vi "XW_file_info.vi"(0 "Instrument type":T1=enum."Cross wire angle", 1 "Ch No":i16) -> (2 "Filename":path, 3 "resulting string":string, 4 "File Exists?":bool)   [LabVIEW 2010]
uses:
  Controls/Cal_Inst_type.ctl
  Globals/Constants_global.vi
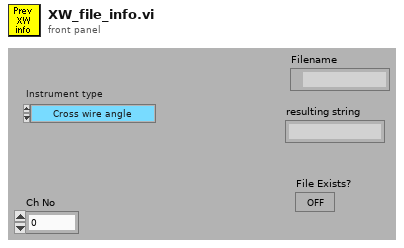
[diagram p1: front panel]
types:
  T1 = typedef "Cal_Inst_type.ctl" = enum16{"Propeller anemometer", "Pressure Transducer", "Hot wire", "Cross wire velocity", "Cross wire angle", "Generic Linear", "Generic Polynomial", "Generic BackPoly", "Fast FID", "Thermocouple", "Cold wire", "Pulsed Wire"}
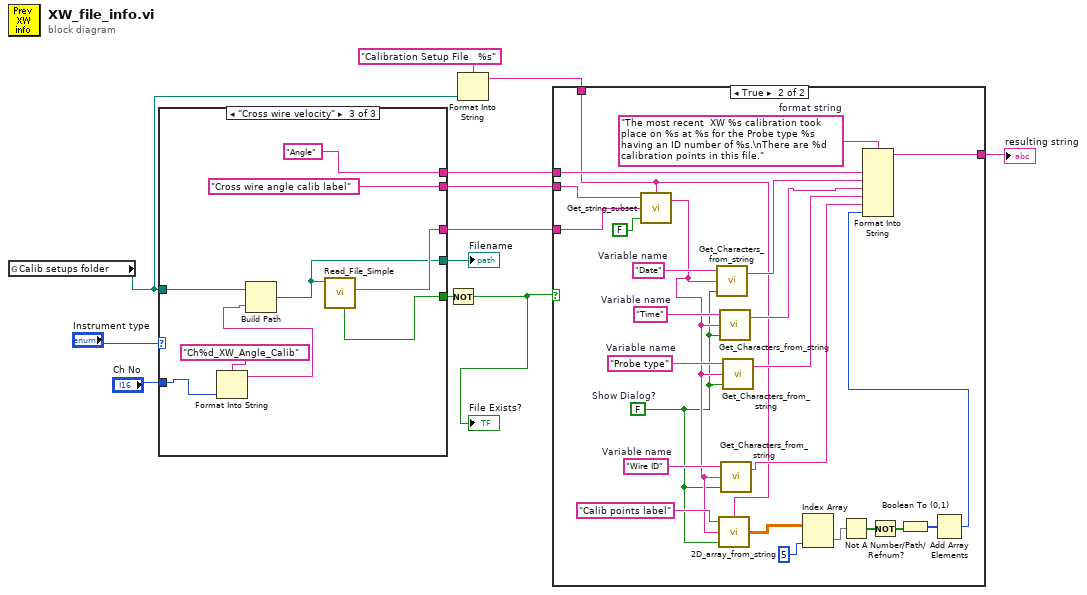
[diagram p0: block diagram]
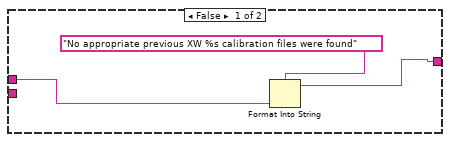
[diagram p2: hidden frame]
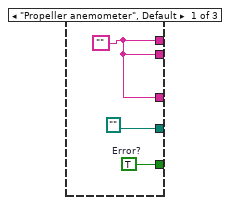
[diagram p3: hidden frame]
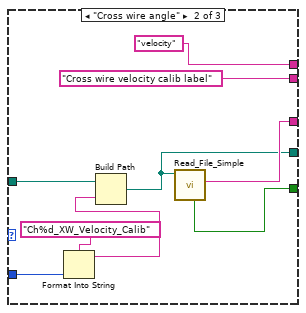
[diagram p4: hidden frame]
diagram:
  n1 = global read "Constants_global.vi" "Calib setups folder"() -> (w2:path)
  n2 = case shown="\"Cross wire velocity\"" "Instrument type" {
    tunnel: w2 -> [_ w24 w33]
    tunnel: [w15 w23 w32] -> w11
    tunnel: [w14 "Cross wire velocity calib label" "Cross wire angle calib label"] -> w9
    tunnel: [w14 w21 w30] -> w8
    tunnel: [w14 "velocity" "Angle"] -> w7
    tunnel: [path "" w19 w28] -> w5
    tunnel: "Ch No" -> [_ w17 w26]
    frame "Propeller anemometer", Default {
      w14 = ""
      w15 = TRUE  # Error?
    }
    frame "Cross wire angle" {
      n3 = Format Into String(format string="Ch%d_XW_Velocity_Calib", w17) -> (resulting string=w16:string)  [unwired: 2 in, 1 out]
      n4 = Build Path(base path=w24, name or relative path=w16) -> (appended path=w19:path)
      n5 = call "Read_File_Simple.vi"("Filename"=w19) -> ("Error?"=w23:bool, "string"=w21:string)  [unwired: 2 in, 6 out]
    }
    frame "Cross wire velocity" {
      n6 = Format Into String(format string="Ch%d_XW_Angle_Calib", w26) -> (resulting string=w25:string)  [unwired: 2 in, 1 out]
      n7 = Build Path(base path=w33, name or relative path=w25) -> (appended path=w28:path)
      n8 = call "Read_File_Simple.vi"("Filename"=w28) -> ("Error?"=w32:bool, "string"=w30:string)  [unwired: 2 in, 6 out]
    }
  }
  "Filename" <- w5
  n9 = Not(x=w11) -> (.not. x?=w10:bool)
  "File Exists?" <- w10
  n10 = Format Into String(format string="Calibration Setup File   %s", w2) -> (resulting string=w1:string)  [unwired: 2 in, 1 out]
  n11 = case shown="True" w10 {
    tunnel: w9 -> [_ w60]
    tunnel: w8 -> [_ w59]
    tunnel: w7 -> [w35 w55]
    tunnel: [w34 w52] -> w6
    tunnel: w1 -> [_ w37]
    frame False {
      n12 = Format Into String(format string="No appropriate previous XW %s calibration files were found", w35) -> (resulting string=w34:string)  [unwired: 2 in, 1 out]
    }
    frame True {
      w44 = "Time"  # Variable name
      w53 = "Wire ID"  # Variable name
      w54 = "The most recent  XW %s calibration took place on %s at %s for the Probe type %s having an ID number of %s.\nThere are %d calibration points in this file."  # format string
      w42 = FALSE  # Show Dialog?
      w57 = "Probe type"  # Variable name
      w58 = "Date"  # Variable name
      n13 = call "Get_string_subset.vi"("String Name"=w37, "Show Dialog?"=FALSE, "String to split"=w59, "File Label"=w60) -> ("Output string"=w43:string)  [unwired: 1 out]
      n14 = call "Get_Characters_from_string.vi"("Show Dialog?"=w42, "Input string"=w43, "Variable name"=w58) -> ("Value"=w56:string)  [unwired: 1 out]
      n15 = call "2D_array_from_string.vi"("String Name"=w37, "Show Dialog?"=w42, "Input string"=w43, "Array title"="Calib points label") -> ("2D data array"=w50:dbl[][])
      n16 = call "Get_Characters_from_string.vi"("Show Dialog?"=w42, "Input string"=w43, "Variable name"=w44) -> ("Value"=w41:string)  [unwired: 1 out]
      n17 = call "Get_Characters_from_string.vi"("Show Dialog?"=w42, "Input string"=w43, "Variable name"=w53) -> ("Value"=w39:string)  [unwired: 1 out]
      n18 = call "Get_Characters_from_string.vi"("Show Dialog?"=w42, "Input string"=w43, "Variable name"=w57) -> ("Value"=w40:string)  [unwired: 1 out]
      n19 = Index Array(array=w50, index (col)=5 ("Index")) -> (element=w48:dbl[])  [unwired: 1 in]
      n20 = Not A Number/Path/Refnum?(number/path/refnum=w48) -> (NaN/Path/Refnum?=w47:bool[])
      n21 = Not(x=w47) -> (.not. x?=w46:bool[])
      n22 = Boolean To (0,1)(Boolean=w46) -> (0, 1=w45:i16[])
      n23 = Add Array Elements(numeric array=w45) -> (sum=w38:i16)
      n24 = Format Into String(format string=w54, w55, w56, w41, w40, w39, w38) -> (resulting string=w52:string)  [unwired: 2 in, 1 out]
    }
  }
  "resulting string" <- w6
